vi "Add.vi"(5 "Create if not Found? (T)":bool=TRUE, 6 "ms Delay (1000)":i32=1000, 7 "Method (Absent)":enum8{"Back", "Front", "Lossy", "Absent"}(ring)=enum."Absent", 8 "error in (no error)":errorcluster, 9 "Start? (T)":bool=TRUE, 10 "Timer Message":string, 11 "Queue in":refnum<queue>) -> (0 "error out":errorcluster, 1 "Created New?":bool, 3 "Queue out":refnum<queue>)   [LabVIEW 2021, in "QueueTimer.lvlib"]
doc: "Add or update a queue timer. Specify the <b>Timer Message</b> to enqueue at every <b>ms Delay</b> if <b>Start?</b> is True. The <b>Method</b> and <b>Timer Message</b> cannot be changed once the timer is created. Recreate the timer to reset the message and method.\n\nUse the <b>List.vi</b> to list all queue timers in memory. Use the <b>Status.vi</b> to return information about the queue timers associated with this queue.\n\nNote: Queue timers are uniquely identified by the `<queue>+<timer_message>`, the same timer message cannot be used for multiple timers. Instead, create unique messages for each timer that call the same case structure.\n\n| Method | Description |\n| --- | --- |\n| Back | Enqueue to back (last out) |\n| Front | Enqueue to front (first out) |\n| Lossy | Enqueue to back, drop front if queue is full |\n| Absent | Enqueue to back only if the element does not exist on the queue (Default) |"
uses:
  QueueTimer.lvlib
  TypeDefs/Timer.ctl
  SubVIs/Daemon.vi
  <vilib>/Utility/error.llb/Error Cluster From Error Code.vi
  <vilib>/ErrorRing/Error Ring.xnode
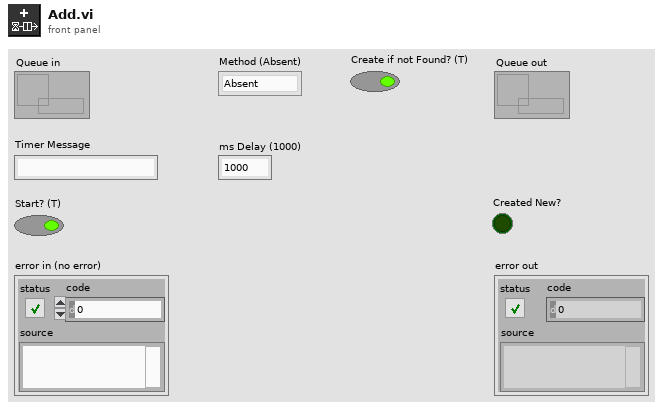
[diagram p1: front panel]
types:
  T1 = typedef "QueueTimer.lvlib/Timer.ctl" = cluster{"Delay":i32, "Start":bool, "Ticks":u32}
  T2 = cluster{"Emit":refnum<queue>, "Time":refnum<data-value>, "Daemon":refnum<vi>}
  T3 = typedef "Queue.lvlib/Timer.ctl" = cluster{"Delay":i32, "Start":bool, "Ticks":u32}
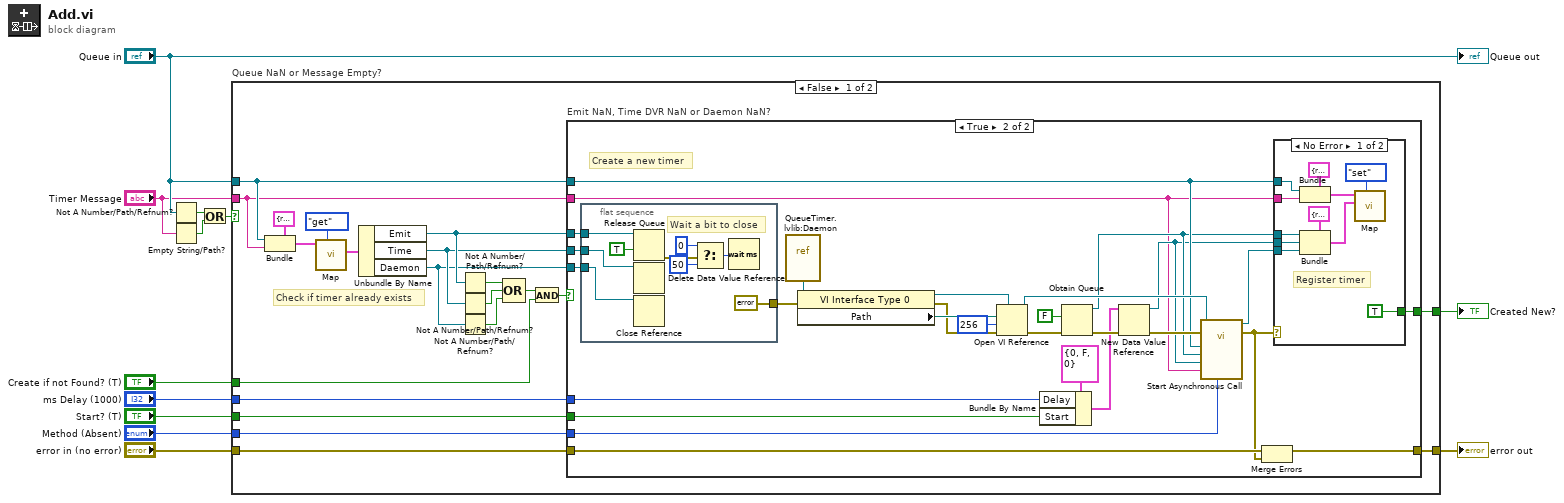
[diagram p0: block diagram]
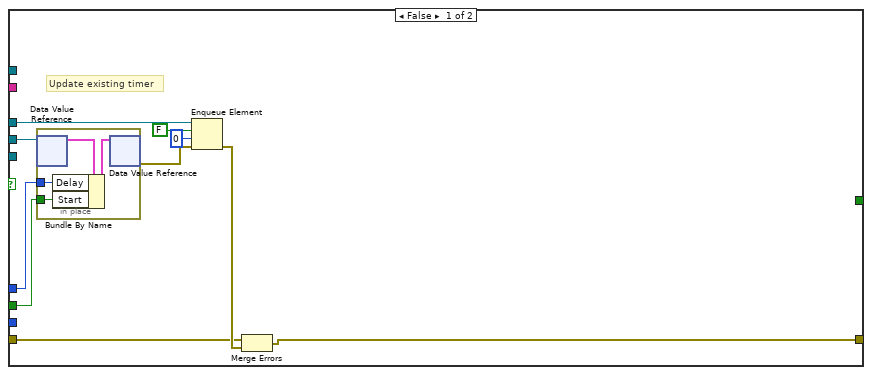
[diagram p2: hidden frame]
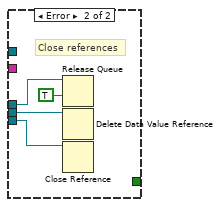
[diagram p3: hidden frame]
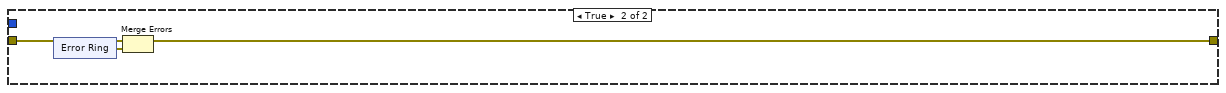
[diagram p4: hidden frame]
diagram:
  n1 = Not A Number/Path/Refnum?(number/path/refnum="Queue in") -> (NaN/Path/Refnum?=w11:bool)
  n2 = Empty String/Path?(string/path="Timer Message") -> (empty?=w12:bool)
  n3 = Or(x=w11, y=w12) -> (x .or. y?=w8:bool)
  n4 = case "Queue NaN or Message Empty?" shown="False" w8 {
    tunnel: "Queue in" -> [w20 _]
    tunnel: "Timer Message" -> [w19 _]
    tunnel: "error in (no error)" -> [w25 w102]
    tunnel: [w24 w101] -> w9
    tunnel: "ms Delay (1000)" -> [w22 _]
    tunnel: "Start? (T)" -> [w21 _]
    tunnel: "Method (Absent)" -> [w18 _]
    tunnel: [w15 _] -> w4
    tunnel: "Create if not Found? (T)" -> [w13 _]
    frame False {
      # "Check if timer already exists"
      n5 = Bundle(cluster=cluster{"Queue":refnum<queue>, "Message":string} {"Queue"=refnum, "Message"=""} ("Timer Id"), "Queue"=w20, "Message"=w19) -> (w23:cluster{"Queue":refnum<queue>, "Message":string})
      n6 = call "Map.vi"("Action"=enum8{"noop", "get", "set", "pop"}."get", "Timer Id"=w23) -> ("Timer out"=w30:T2)  [unwired: 7 in, 2 out]
      n7 = Unbundle By Name(w30) -> ("Emit"=w27:refnum<queue>, "Time"=w26:refnum<data-value>, "Daemon"=w16:refnum<vi>)
      n8 = Not A Number/Path/Refnum?(number/path/refnum=w27) -> (NaN/Path/Refnum?=w32:bool)
      n9 = Not A Number/Path/Refnum?(number/path/refnum=w26) -> (NaN/Path/Refnum?=w31:bool)
      n10 = Not A Number/Path/Refnum?(number/path/refnum=w16) -> (NaN/Path/Refnum?=w17:bool)
      n11 = Compound Arithmetic op=OR(w32, w31, w17) -> (w28:bool)
      n12 = And(x=w28, y=w13) -> (x .and. y?=w14:bool)
      n13 = case "Emit NaN, Time DVR NaN or Daemon NaN?" shown="True" w14 {
        tunnel: w27 -> [w35 w73]
        tunnel: w26 -> [w43 w72]
        tunnel: w25 -> [w39 w52]
        tunnel: [w38 w51] -> w24
        tunnel: w22 -> [w37 w69]
        tunnel: w21 -> [w36 w68]
        tunnel: w20 -> [_ w59]
        tunnel: w19 -> [_ w56]
        tunnel: w18 -> [_ w55]
        tunnel: w16 -> [_ w49]
        tunnel: [_ w48] -> w15
        frame False {
          # "Update existing timer"
          n14 = in-place {
            in-place-border: w37 -> [w45]
            in-place-border: w36 -> [w44]
            n15 = in-place-dvr #1(w43) -> (w47:T3)  [unwired: 1 out]
            n16 = Bundle By Name(cluster=w47, "Delay"=w45, "Start"=w44) -> (w46:T3)
            n17 = in-place-dvr #1(w46) -> (w41:errorcluster)  [unwired: 1 out]
          }
          n18 = Enqueue Element(queue=w35, element=FALSE, timeout in ms (-1)=0, error in (no error)=w41) -> (error out=w40:errorcluster)  [unwired: 2 out]
          n19 = Merge Errors(w39, w40) -> (w38:errorcluster)
        }
        frame True {
          # "Create a new timer"
          n20 = flat-sequence {
            tunnel: w73 -> [w84]
            tunnel: w72 -> [w82]
            tunnel: [errorcluster {"status"=FALSE, "code"=0, "source"=""} ("error in (no error)")] -> w53
            tunnel: w49 -> [w80]
            frame #0 {
              # "Wait a bit to close"
              n21 = Release Queue(queue=w84, force destroy? (F)=TRUE) -> (error out=w79:errorcluster)  [unwired: 1 in, 2 out]
              n22 = Delete Data Value Reference(data value reference=w82) -> ()  [unwired: 1 in, 2 out]
              n23 = Close Reference(reference=w80) -> ()  [unwired: 1 in, 1 out]
              n24 = Select(t=u32 0 ("milliseconds to wait"), s=w79, f=u32 50 ("milliseconds to wait")) -> (s? t:f=w76:u32)
              n25 = Wait (ms)(milliseconds to wait=w76) -> ()  [unwired: 1 out]
            }
          }
          n26 = vi-ref "QueueTimer.lvlib:Daemon.vi"() -> (w67:refnum<vi>)
          n27 = property class="VI Interface Type 0"(reference=w67, error in=w53) -> (reference out=w64:refnum<vi>, error out=w65:errorcluster, "Path"=w66:path)
          n28 = Open VI Reference(type specifier VI Refnum (for type only)=w64, vi path=w66, options=256, error in (no error)=w65) -> (vi reference=w60:refnum<vi>, error out=w62:errorcluster)  [unwired: 2 in]
          n29 = Bundle By Name(cluster=T1 {"Delay"=0, "Start"=FALSE, "Ticks"=0} ("Timer"), "Delay"=w69, "Start"=w68) -> (w70:T1)
          n30 = Obtain Queue(element data type=FALSE, error in (no error)=w62) -> (queue out=w58:refnum<queue>, error out=w71:errorcluster)  [unwired: 3 in, 1 out]
          n31 = New Data Value Reference(data value=w70, error in=w71) -> (data value reference=w57:refnum<data-value>, error out=w61:errorcluster)
          n32 = call-by-ref "Start Asynchronous Call"(reference=w60, error in=w61, "Method"=w55, "Message"=w56, "Time"=w57, "Emit"=w58, "Queue"=w59) -> (reference out=w54:refnum<vi>, error out=w50:errorcluster)  [unwired: 7 in]
          n33 = Merge Errors(w52, w50) -> (w51:errorcluster)
          n34 = case shown="No Error" w50 {
            tunnel: w59 -> [w90 _]
            tunnel: w58 -> [w89 w99]
            tunnel: w57 -> [w88 w97]
            tunnel: w56 -> [w87 _]
            tunnel: w54 -> [w86 w96]
            tunnel: [TRUE _] -> w48
            frame No Error {
              # "Register timer"
              n35 = Bundle(cluster=cluster{"Queue":refnum<queue>, "Message":string} {"Queue"=refnum, "Message"=""} ("Timer Id"), "Queue"=w90, "Message"=w87) -> (w91:cluster{"Queue":refnum<queue>, "Message":string})
              n36 = Bundle(cluster=T2 {"Emit"=refnum, "Time"=refnum, "Daemon"=refnum} ("Timer in"), "Emit"=w89, "Time"=w88, "Daemon"=w86) -> (w93:T2)
              n37 = call "Map.vi"("Action"=enum8{"noop", "get", "set", "pop"}."set", "Timer in"=w93, "Timer Id"=w91) -> ()  [unwired: 6 in, 3 out]
            }
            frame Error {
              # "Close references"
              n38 = Release Queue(queue=w99, force destroy? (F)=TRUE) -> ()  [unwired: 1 in, 3 out]
              n39 = Delete Data Value Reference(data value reference=w97) -> ()  [unwired: 1 in, 2 out]
              n40 = Close Reference(reference=w96) -> ()  [unwired: 1 in, 1 out]
            }
          }
        }
      }
    }
    frame True {
      n41 = xnode "Error Ring"() -> ("error out"=w100:errorcluster)
      n42 = Merge Errors(w102, w100) -> (w101:errorcluster)
    }
  }
  "error out" <- w9
  "Created New?" <- w4
  "Queue out" <- "Queue in"
